vi "myRIO_BRig_RT_comm_webdav_uploadFile__data__v2.vi"(8 "input_error":errorcluster, 9 "input_fileName_prefix":string, 10 "input_fileName":string="dataTrial", 11 "input_hSession":T1) -> (0 "output_error":errorcluster, 2 "output_IsentFile_exp":bool, 3 "output_hSession":T1)   [LabVIEW 2014]
uses:
  <vilib>/WebDAVClient/Advanced/SessionHandle.ctl
  <vilib>/WebDAVClient/Advanced/Put File.vi
  <vilib>/WebDAVClient/NI_WebDAV.lvlib
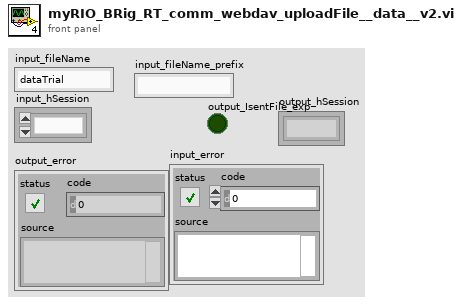
[diagram p1: front panel]
types:
  T1 = typedef "NI_WebDAV.lvlib/SessionHandle.ctl" = refnum<k1>
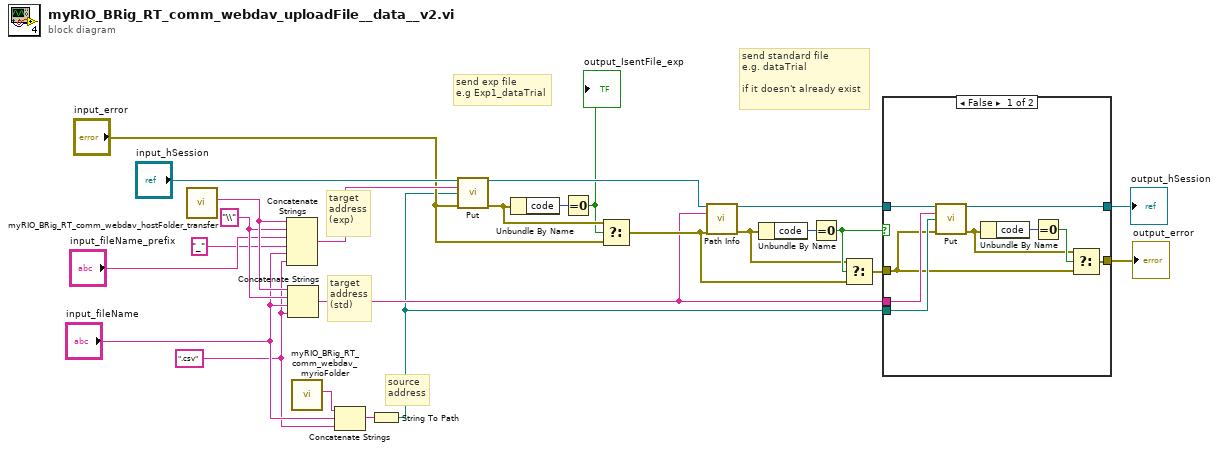
[diagram p0: block diagram]
diagram:
  w21 = "\\" ("string")
  w17 = ".csv" ("string")
  # "source\naddress"
  # "target\naddress\n(std)"
  # "target\naddress\n(exp)"
  # "send exp file\ne.g Exp1_dataTrial"
  # "send standard file\ne.g. dataTrial\n\nif it doesn't already exist"
  n1 = call "myRIO_BRig_RT_comm_webdav_hostFolder_transfer.vi"() -> ("output_HostFolder"=w22:string)  [unwired: 11 in]
  n2 = Concatenate Strings(w22, w21, "input_fileName_prefix", "_" ("string"), "input_fileName", w17) -> (w23:string)
  n3 = Concatenate Strings(w22, w21, "input_fileName", w17) -> (w5:string)
  n4 = call "myRIO_BRig_RT_comm_webdav_myrioFolder.vi"() -> ("output_myrioFolder"=w24:string)  [unwired: 11 in]
  n5 = Concatenate Strings(w24, "input_fileName", w17) -> (w25:string)
  n6 = String To Path(string=w25) -> (path=w4:path)
  n7 = call-poly <vilib>:"Put.vi"("session handle"="input_hSession", "relative uri"=w23, "local file path"=w4, "error in (no error)"="input_error") -> ("session handle out"=w12:T1, "error out"=w14:errorcluster)  [unwired: 9 in, 1 out]
  n8 = Unbundle By Name(w14) -> ("code"=w16:i32)
  n9 = Equal To 0?(x=w16) -> (x = 0?=w3:bool)
  "output_IsentFile_exp" <- w3
  n10 = Select(t=w14, s=w3, f="input_error") -> (s? t:f=w8:errorcluster)
  n11 = call <vilib>:"Path Info.vi"("session handle"=w12, "relative uri"=w5, "error in (no error)"=w8) -> ("session handle out"=w6:T1, "error out"=w9:errorcluster)  [unwired: 9 in, 2 out]
  n12 = Unbundle By Name(w9) -> ("code"=w11:i32)
  n13 = Equal To 0?(x=w11) -> (x = 0?=w10:bool)
  n14 = Select(t=w9, s=w10, f=w8) -> (s? t:f=w7:errorcluster)
  n15 = case shown="False" w10 {
    tunnel: w7 -> [w28 w36]
    tunnel: w6 -> [w34 w35]
    tunnel: w5 -> [w32 _]
    tunnel: w4 -> [w33 _]
    tunnel: [w27 w36] -> w1
    tunnel: [w26 w35] -> w2
    frame False {
      n16 = call-poly <vilib>:"Put.vi"("session handle"=w34, "relative uri"=w32, "local file path"=w33, "error in (no error)"=w28) -> ("session handle out"=w26:T1, "error out"=w29:errorcluster)  [unwired: 9 in, 1 out]
      n17 = Unbundle By Name(w29) -> ("code"=w31:i32)
      n18 = Equal To 0?(x=w31) -> (x = 0?=w30:bool)
      n19 = Select(t=w29, s=w30, f=w28) -> (s? t:f=w27:errorcluster)
    }
    frame True {
    }
  }
  "output_error" <- w1
  "output_hSession" <- w2
